vi "integrator.vi"(11 "y":fxp<+/-,24,24>) -> (3 "Numeric":fxp<+/-,24,24>)   [LabVIEW 2013]
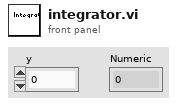
[diagram p1: front panel]
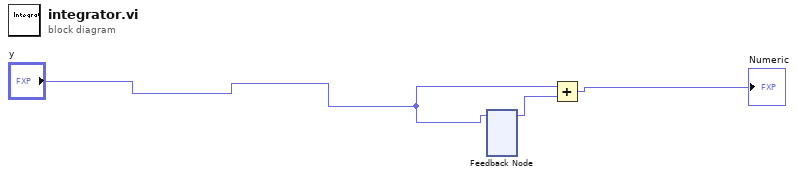
[diagram p0: block diagram]
diagram:
  n1 = feedback #1() -> (w3:fxp<+/-,24,24>)  [unwired: 1 in]
  n2 = feedback-in #1("y") -> ()
  n3 = Add(x="y", y=w3) -> (x+y=→"Numeric":fxp<+/-,24,24>)
